vi "Read RoomParams.vi"(8 "error in (no error)":errorcluster, 11 "Room":refnum<class "Room.lvclass">) -> (0 "error out":errorcluster, 2 "RoomParams":T1, 3 "Room":refnum<class "Room.lvclass">)   [LabVIEW 2020, in "Room.lvclass"]
uses:
  Room.lvclass
  TypeDef/RoomParams.ctl
  Room.lvclass/Room.ctl
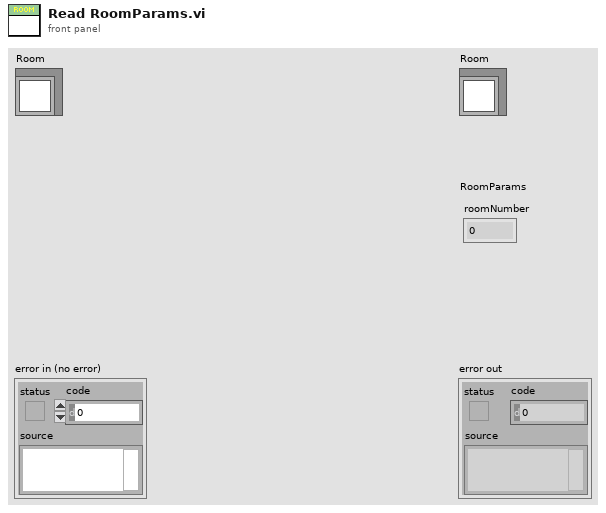
[diagram p1: front panel]
types:
  T1 = typedef "Room.lvclass/RoomParams.ctl" = cluster{"roomNumber":i32}
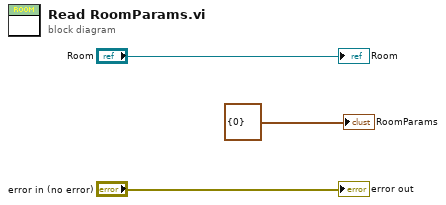
[diagram p0: block diagram]
diagram:
  "error out" <- "error in (no error)"
  "Room" <- "Room"
  "RoomParams" <- T1 {"roomNumber"=0} ("<ClassName>Params")
